vi "Set Active Plugins.vi"(10 "Active Plugins":bool[](array[boolean]), 11 "Framework State in":refnum<class "Framework State.lvclass">) -> (3 "Framework State out":refnum<class "Framework State.lvclass">)   [LabVIEW 2017, in "Data Sharing Framework Engine.lvlib" / "Framework State.lvclass"]
uses:
  Framework State.lvclass
  Framework State.lvclass/Framework State.ctl
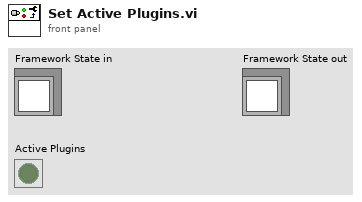
[diagram p1: front panel]
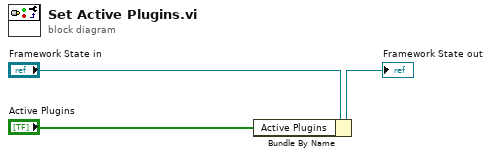
[diagram p0: block diagram]
diagram:
  n1 = Bundle By Name(cluster="Framework State in", "Active Plugins"="Active Plugins") -> (→"Framework State out":refnum<class "Framework State.lvclass">)
